vi "Cost.vi"(8 "error in (no error)":errorcluster, 11 "Decaf in":refnum<class "Decaf.lvclass">) -> (0 "error out":errorcluster, 2 "Cost":dbl, 3 "Decaf out":refnum<class "Decaf.lvclass">)   [LabVIEW 2020, in "Decaf.lvclass"]
uses:
  Decaf.lvclass
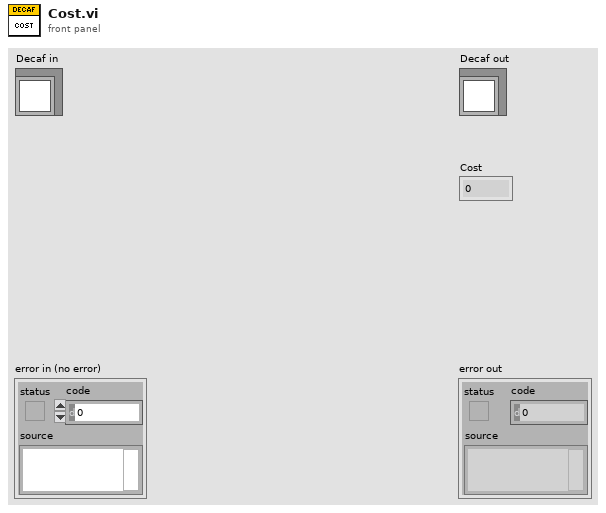
[diagram p1: front panel]
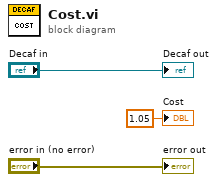
[diagram p0: block diagram]
diagram:
  "error out" <- "error in (no error)"
  "Decaf out" <- "Decaf in"
  "Cost" <- 1.05 ("Cost")
